vi "z encoding equals.vi"(8 "error in (no error)":errorcluster, 10 "other":cluster{}, 11 "this_":cluster{}) -> (0 "error out":errorcluster, 3 "function return":bool)   [LabVIEW 2021, in "zenohc.lvlib"]
doc: "bool z_encoding_equals(const struct z_loaned_encoding_t *this_,\n const struct z_loaned_encoding_t *other);"
uses:
  zenohc.lvlib
  zenohc.dll
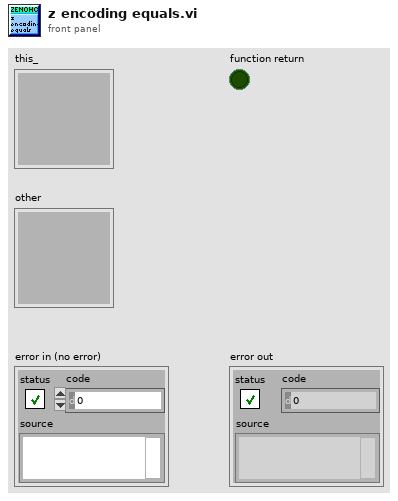
[diagram p1: front panel]
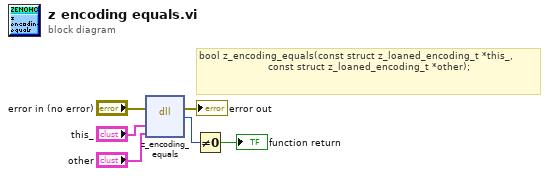
[diagram p0: block diagram]
diagram:
  # "bool z_encoding_equals(const struct z_loaned_encoding_t *this_,\n                       const struct z_loaned_encoding_t *other);"
  n1 = dll-call lib="D:/dev/zenoh_labview/zenohc/zenohc.*" fn="z_encoding_equals"(error in="error in (no error)", "this_"="this_", "other"="other") -> (error out=→"error out":errorcluster, w5:u8)  [unwired: 4 in, 1 out]
  n2 = Not Equal To 0?(x=w5) -> (x != 0?=→"function return":bool)
